vi "Wait_ms.vi"(3 "[IN] Suspend ms":u32, 5 "error IN":errorcluster) -> (2 "error OUT":errorcluster)   [LabVIEW 2020]
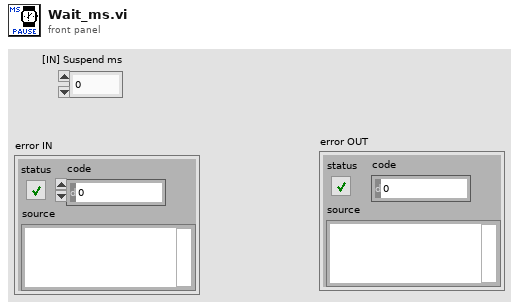
[diagram p1: front panel]
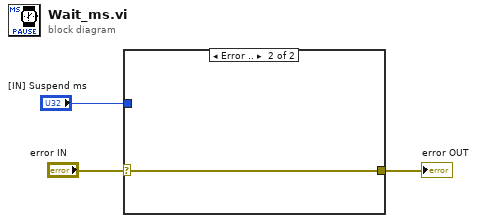
[diagram p0: block diagram]
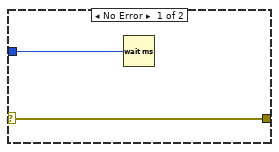
[diagram p2: hidden frame]
diagram:
  n1 = case shown="Error .." "error IN" {
    selector: "error IN" -> [w5 w6]
    tunnel: [w5 w6] -> w2
    tunnel: "[IN] Suspend ms" -> [w4 _]
    frame No Error {
      n2 = Wait (ms)(milliseconds to wait=w4) -> ()  [unwired: 1 out]
    }
    frame Error {
    }
  }
  "error OUT" <- w2
